vi "数据处理.vi"(9 "输入数组":dbl[](array[numeric]), 11 "读取数据":dbl[](array[numeric])) -> (1 "输出数组":dbl[](array[numeric]), 2 "mean":dbl caption="均值" format="%0.2f", 3 "当前温度":dbl)   [LabVIEW 2020]
uses:
  <vilib>/Analysis/baseanly.llb/Mean (DBL).vi
  <vilib>/Analysis/NI_AALBase.lvlib
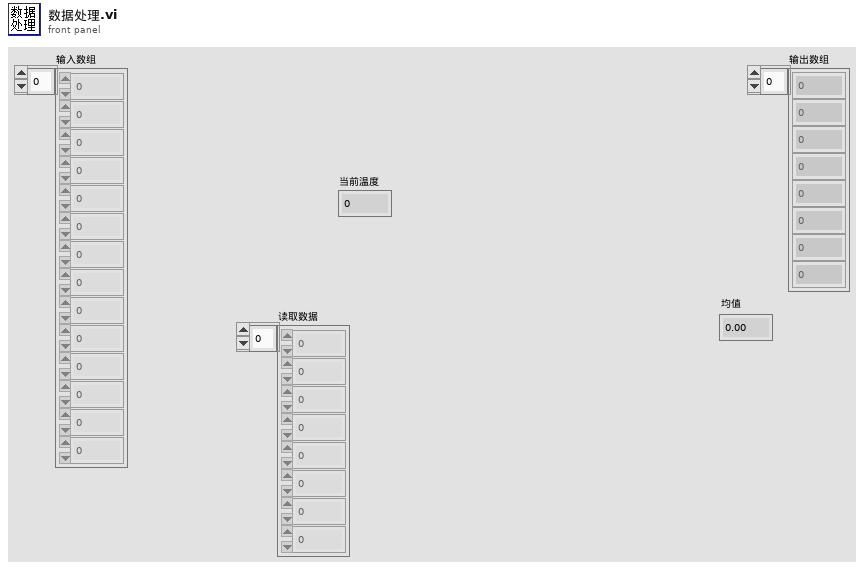
[diagram p1: front panel]
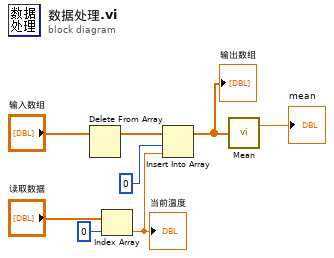
[diagram p0: block diagram]
diagram:
  n1 = Delete From Array(array="输入数组") -> (array with subset deleted=w5:dbl[])  [unwired: 2 in, 1 out]
  n2 = Index Array(array="读取数据", index=0 ("索引")) -> (element=w4:dbl)
  "当前温度" <- w4
  n3 = Insert Into Array(array=w5, index=0 ("索引"), new element=w4) -> (w2:dbl[])
  "输出数组" <- w2
  n4 = call-poly <vilib>:"Mean.vi"("X"=w2) -> ("mean"=→"mean":dbl)  [unwired: 1 out]
